vi "HEWH ANSI Get Rates.vi"(0 "ANSI Rate in":T3, 1 "Test Type - Rate":string(combo)="Rate", 5 "CO CO2 Data Array":string[][](array[string]), 7 "Gas Measurment Data":T2, 9 "Inficon Data - ALL":T1, 11 "error in (no error)":errorcluster, 12 "Software Elapsed Time":dbl format="%<%H:%M:%S>t") -> (3 "ANSI Display 1":string, 4 "ANSI Rate out":T3, 8 "Rate Outputs":string[][](array[string]), 14 "Test Complete":bool, 15 "error out":errorcluster)   [LabVIEW 2020]
uses:
  HEWH ANSI Rate.ctl
  Drivers/Alicat LabVIEW Drivers 2v1/Sub-VIs/Data Cluster.ctl
  Drivers/Inficon Transmitter/Type Definitions/Inficon Data.ctl
panel:
  out "Raw Timer Output":dbl format="%<%H:%M:%S>t"
  # "Natural Gas"
  # "Propane"
  # "Totalizer Timer"
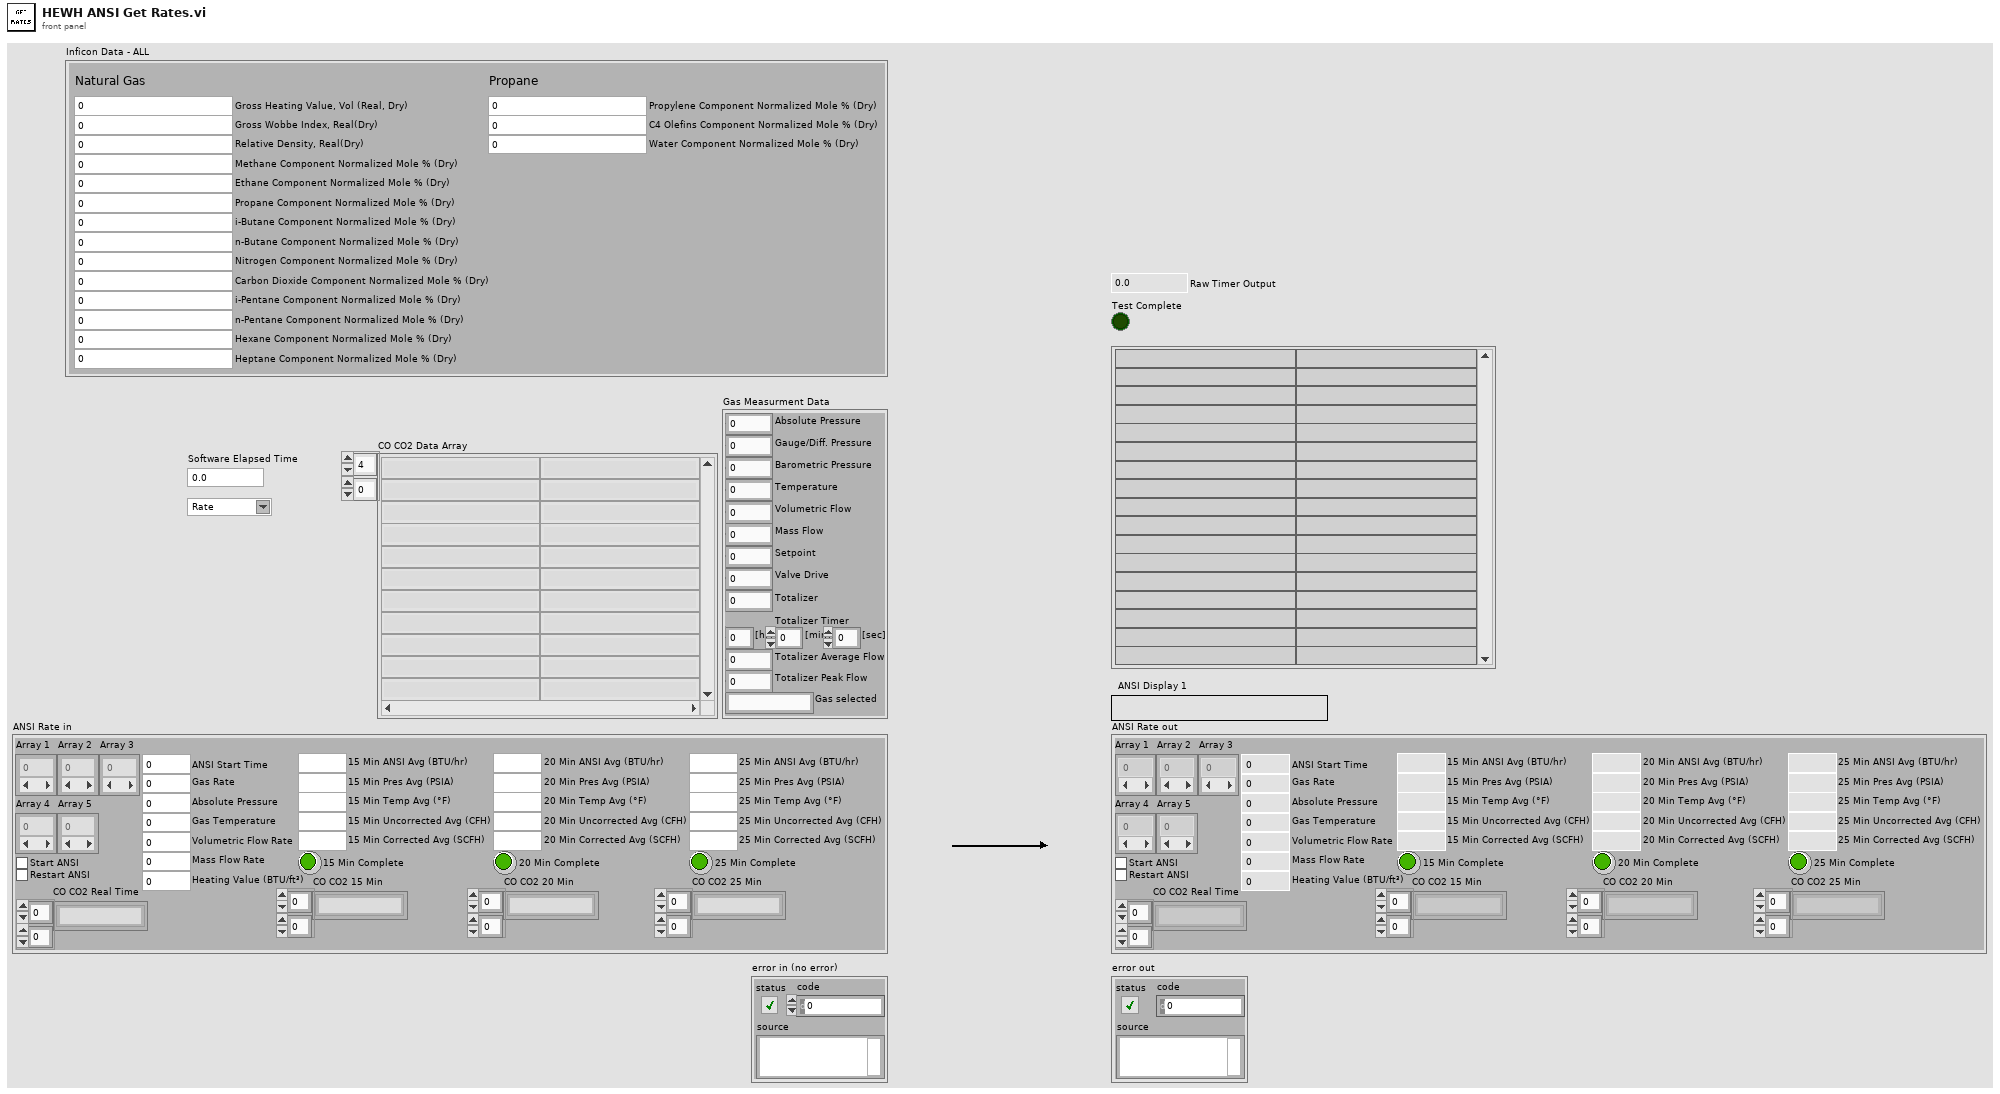
[diagram p1: front panel]
types:
  T1 = typedef "Inficon Data.ctl" = cluster{"Gross Heating Value, Vol (Real, Dry)":dbl, "Nitrogen Component Normalized Mole % (Dry)":dbl, "Methane Component Normalized Mole % (Dry)":dbl, "Carbon Dioxide Component Normalized Mole % (Dry)":dbl, "Ethane Component Normalized Mole % (Dry)":dbl, "Propane Component Normalized Mole % (Dry)":dbl, "i-Pentane Component Normalized Mole % (Dry)":dbl, "i-Butane Component Normalized Mole % (Dry)":dbl, "n-Butane Component Normalized Mole % (Dry)":dbl, "n-Pentane Component Normalized Mole % (Dry)":dbl, "Hexane Component Normalized Mole % (Dry)":dbl, "Heptane Component Normalized Mole % (Dry)":dbl, "Gross Wobbe Index, Real(Dry)":dbl, "Relative Density, Real(Dry)":dbl, "Propylene Component Normalized Mole % (Dry)":dbl, "C4 Olefins Component Normalized Mole % (Dry)":dbl, "Water Component Normalized Mole % (Dry)":dbl}
  T2 = typedef "Data Cluster.ctl" = cluster{"Absolute Pressure":dbl, "Gauge/Diff. Pressure":dbl, "Barometric Pressure":dbl, "Temperature":dbl, "Volumetric Flow":dbl, "Mass Flow":dbl, "Setpoint":dbl, "Valve Drive":dbl, "Totalizer":dbl, "[hr]":dbl, "[min]":dbl, "[sec]":dbl, "Totalizer Average Flow":dbl, "Totalizer Peak Flow":dbl, "Gas selected":string}
  T3 = typedef "HEWH ANSI Rate.ctl" = cluster{"Array 1":dbl[], "Array 3":dbl[], "Array 2":dbl[], "Start ANSI":bool, "ANSI Start Time":dbl, "Restart ANSI":bool, "15 Min ANSI Avg (BTU/hr)":dbl, "20 Min ANSI Avg (BTU/hr)":dbl, "25 Min ANSI Avg (BTU/hr)":dbl, "Absolute Pressure":dbl, "Gas Temperature":dbl, "Volumetric Flow Rate":dbl, "Mass Flow Rate":dbl, "Array 4":dbl[], "Array 5":dbl[], "Gas Rate":dbl, "15 Min Pres Avg (PSIA)":dbl, "20 Min Pres Avg (PSIA)":dbl, "25 Min Pres Avg (PSIA)":dbl, "15 Min Temp Avg (°F) ":dbl, "20 Min Temp Avg (°F)":dbl, "25 Min Temp Avg (°F)":dbl, "15 Min Uncorrected Avg (CFH)":dbl, "20 Min Uncorrected Avg (CFH)":dbl, "25 Min Uncorrected Avg (CFH)":dbl, "15 Min Corrected Avg (SCFH)":dbl, "20 Min Corrected Avg (SCFH)":dbl, "25 Min Corrected Avg (SCFH)":dbl, "15 Min Complete":bool, "20 Min Complete":bool, "25 Min Complete":bool, "Heating Value (BTU/ft³)":dbl, "CO CO2 15 Min":string[][], "CO CO2 20 Min":string[][], "CO CO2 25 Min":string[][], "CO CO2 Real Time":string[][]}
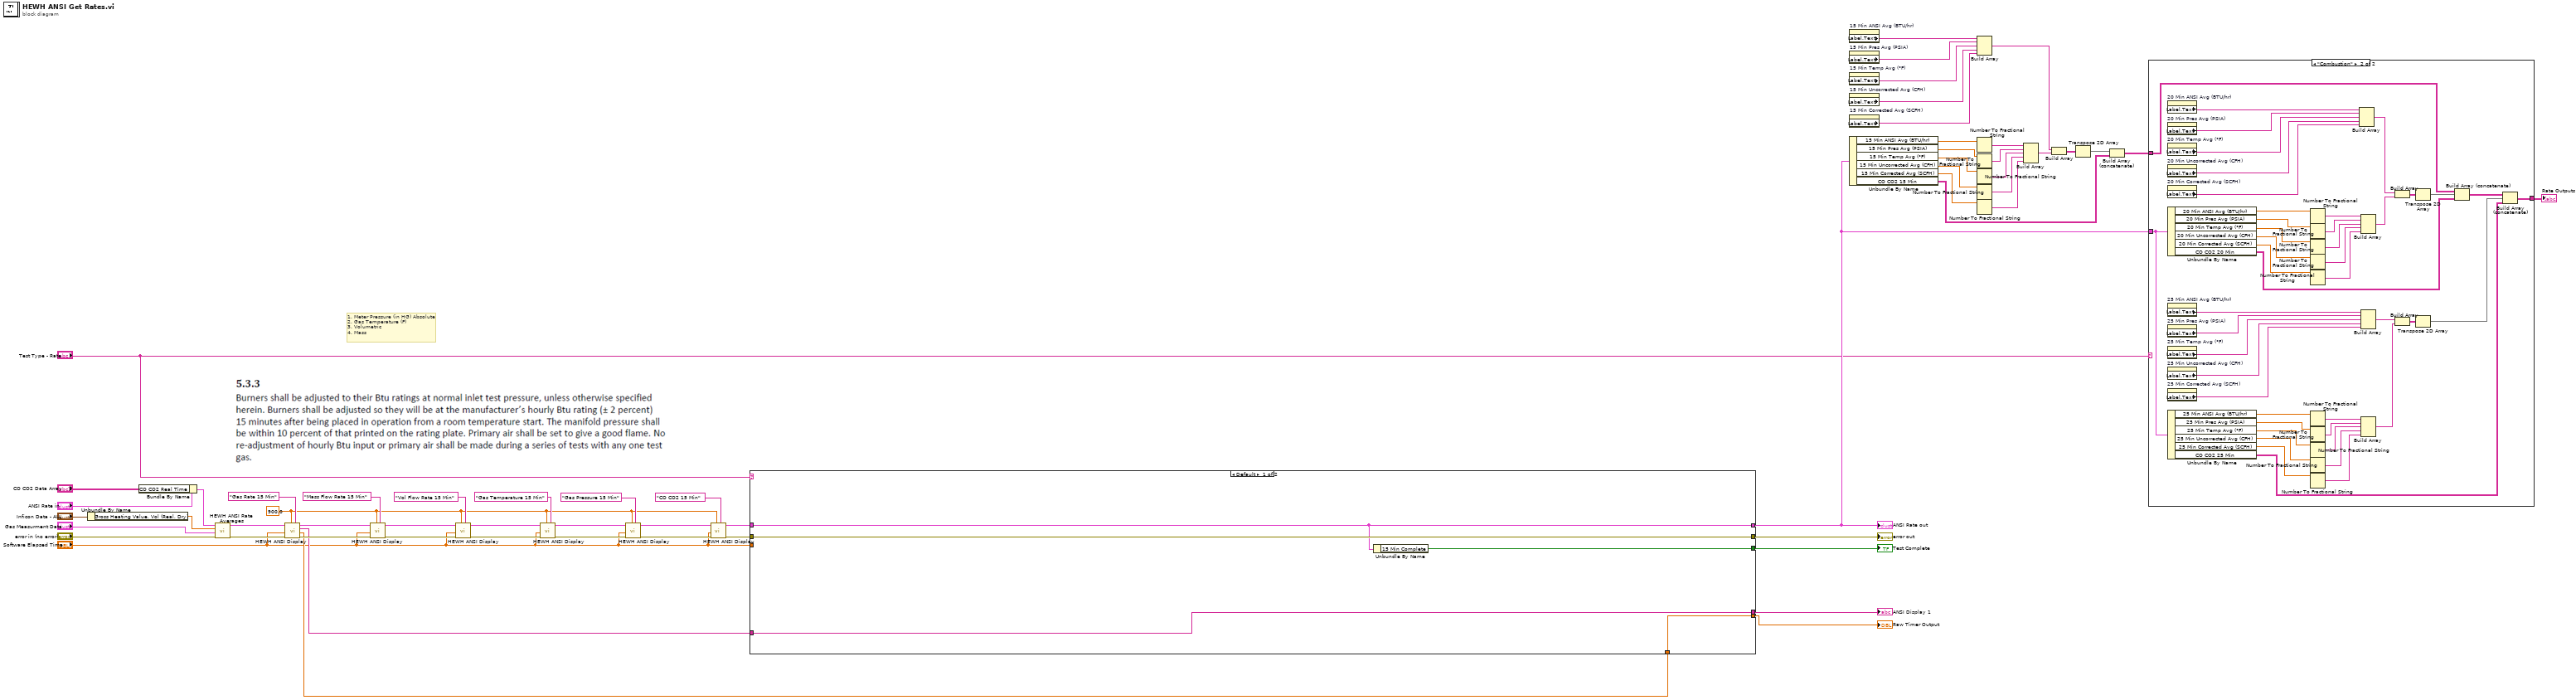
[diagram p0: block diagram]
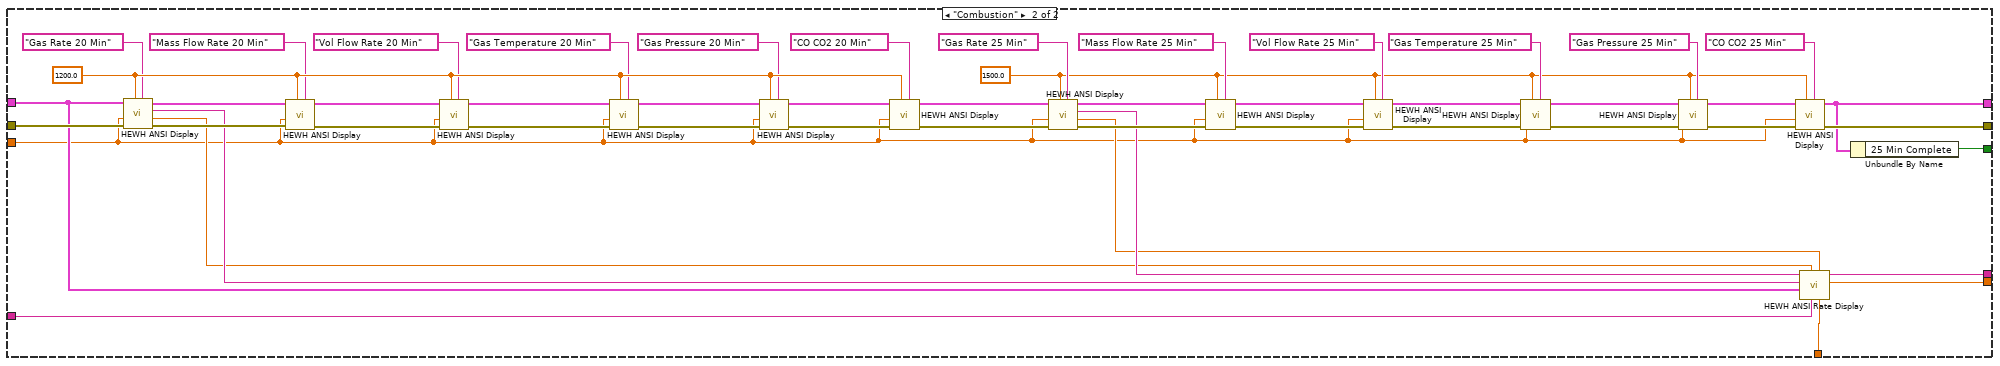
[diagram p3: hidden frame]
diagram:
  w11 = 900.0 ("Stop Timer")
  # "1. Meter Pressure (in HG) Absolute\n2. Gas Temperature (F)\n3. Volumetric\n4. Mass"
  n1 = Unbundle By Name("Inficon Data - ALL") -> ("Gross Heating Value, Vol (Real, Dry)"=w1:dbl)
  n2 = Bundle By Name(cluster="ANSI Rate in", "CO CO2 Real Time"="CO CO2 Data Array") -> (w9:T3)
  n3 = call "HEWH ANSI Rate Averages.vi"("error in (no error)"="error in (no error)", "Gas Measurment Data"="Gas Measurment Data", "Gross Heating Value, Vol (Real, Dry)"=w1, "ANSI Rate in"=w9) -> ("error out"=w57:errorcluster, "ANSI Rate out"=w56:T3)  [unwired: 6 in]
  n4 = call "HEWH ANSI Display.vi"("Calculation Type"="Gas Rate 15 Min", "Stop Timer"=w11, "Error In"=w57, "Software Elapsed Time"="Software Elapsed Time", "ANSI Rate In"=w56) -> ("Error Out"=w51:errorcluster, "Raw Timer"=w22:dbl, "ANSI Display"=w24:string, "ANSI Rate Out"=w55:T3)  [unwired: 3 in]
  n5 = call "HEWH ANSI Display.vi"("Calculation Type"="Mass Flow Rate 15 Min", "Stop Timer"=w11, "Error In"=w51, "Software Elapsed Time"="Software Elapsed Time", "ANSI Rate In"=w55) -> ("Error Out"=w50:errorcluster, "ANSI Rate Out"=w54:T3)  [unwired: 3 in, 2 out]
  n6 = call "HEWH ANSI Display.vi"("Calculation Type"="Vol Flow Rate 15 Min", "Stop Timer"=w11, "Error In"=w50, "Software Elapsed Time"="Software Elapsed Time", "ANSI Rate In"=w54) -> ("Error Out"=w49:errorcluster, "ANSI Rate Out"=w53:T3)  [unwired: 3 in, 2 out]
  n7 = call "HEWH ANSI Display.vi"("Calculation Type"="Gas Temperature 15 Min", "Stop Timer"=w11, "Error In"=w49, "Software Elapsed Time"="Software Elapsed Time", "ANSI Rate In"=w53) -> ("Error Out"=w48:errorcluster, "ANSI Rate Out"=w52:T3)  [unwired: 3 in, 2 out]
  n8 = call "HEWH ANSI Display.vi"("Calculation Type"="Gas Pressure 15 Min", "Stop Timer"=w11, "Error In"=w48, "Software Elapsed Time"="Software Elapsed Time", "ANSI Rate In"=w52) -> ("Error Out"=w13:errorcluster, "ANSI Rate Out"=w15:T3)  [unwired: 3 in, 2 out]
  n9 = call "HEWH ANSI Display.vi"("Calculation Type"="CO CO2 15 Min", "Stop Timer"=w11, "Error In"=w13, "Software Elapsed Time"="Software Elapsed Time", "ANSI Rate In"=w15) -> ("Error Out"=w12:errorcluster, "ANSI Rate Out"=w14:T3)  [unwired: 3 in, 2 out]
  n10 = case shown="Default" "Test Type - Rate" {
    tunnel: w12 -> [w64 w114]
    tunnel: w14 -> [w63 w96]
    tunnel: [w64 w70] -> w47
    tunnel: [w63 w68] -> w46
    tunnel: "Software Elapsed Time" -> [_ w66]
    tunnel: [w62 w97] -> w25
    tunnel: w24 -> [w61 w95]
    tunnel: [w61 w94] -> w23
    tunnel: w22 -> [w60 w91]
    tunnel: [w60 w88] -> w3
    frame Default {
      n11 = Unbundle By Name(w63) -> ("15 Min Complete"=w62:bool)
    }
    frame "Combustion" {
      w67 = 1500.0 ("Stop Timer")
      w82 = 1200.0 ("Stop Timer")
      n12 = call "HEWH ANSI Display.vi"("Calculation Type"="Gas Rate 20 Min", "Stop Timer"=w82, "Error In"=w114, "Software Elapsed Time"=w66, "ANSI Rate In"=w96) -> ("Error Out"=w113:errorcluster, "Raw Timer"=w90:dbl, "ANSI Display"=w93:string, "ANSI Rate Out"=w106:T3)  [unwired: 3 in]
      n13 = call "HEWH ANSI Display.vi"("Calculation Type"="Mass Flow Rate 20 Min", "Stop Timer"=w82, "Error In"=w113, "Software Elapsed Time"=w66, "ANSI Rate In"=w106) -> ("Error Out"=w112:errorcluster, "ANSI Rate Out"=w107:T3)  [unwired: 3 in, 2 out]
      n14 = call "HEWH ANSI Display.vi"("Calculation Type"="Vol Flow Rate 20 Min", "Stop Timer"=w82, "Error In"=w112, "Software Elapsed Time"=w66, "ANSI Rate In"=w107) -> ("Error Out"=w111:errorcluster, "ANSI Rate Out"=w108:T3)  [unwired: 3 in, 2 out]
      n15 = call "HEWH ANSI Display.vi"("Calculation Type"="Gas Temperature 20 Min", "Stop Timer"=w82, "Error In"=w111, "Software Elapsed Time"=w66, "ANSI Rate In"=w108) -> ("Error Out"=w110:errorcluster, "ANSI Rate Out"=w109:T3)  [unwired: 3 in, 2 out]
      n16 = call "HEWH ANSI Display.vi"("Calculation Type"="Gas Pressure 20 Min", "Stop Timer"=w82, "Error In"=w110, "Software Elapsed Time"=w66, "ANSI Rate In"=w109) -> ("Error Out"=w84:errorcluster, "ANSI Rate Out"=w87:T3)  [unwired: 3 in, 2 out]
      n17 = call "HEWH ANSI Display.vi"("Calculation Type"="CO CO2 20 Min", "Stop Timer"=w82, "Error In"=w84, "Software Elapsed Time"=w66, "ANSI Rate In"=w87) -> ("Error Out"=w83:errorcluster, "ANSI Rate Out"=w86:T3)  [unwired: 3 in, 2 out]
      n18 = call "HEWH ANSI Display.vi"("Calculation Type"="Gas Rate 25 Min", "Stop Timer"=w67, "Error In"=w83, "Software Elapsed Time"=w66, "ANSI Rate In"=w86) -> ("Error Out"=w105:errorcluster, "Raw Timer"=w89:dbl, "ANSI Display"=w92:string, "ANSI Rate Out"=w101:T3)  [unwired: 3 in]
      n19 = call "HEWH ANSI Display.vi"("Calculation Type"="Mass Flow Rate 25 Min", "Stop Timer"=w67, "Error In"=w105, "Software Elapsed Time"=w66, "ANSI Rate In"=w101) -> ("Error Out"=w104:errorcluster, "ANSI Rate Out"=w100:T3)  [unwired: 3 in, 2 out]
      n20 = call "HEWH ANSI Display.vi"("Calculation Type"="Vol Flow Rate 25 Min", "Stop Timer"=w67, "Error In"=w104, "Software Elapsed Time"=w66, "ANSI Rate In"=w100) -> ("Error Out"=w103:errorcluster, "ANSI Rate Out"=w99:T3)  [unwired: 3 in, 2 out]
      n21 = call "HEWH ANSI Display.vi"("Calculation Type"="Gas Temperature 25 Min", "Stop Timer"=w67, "Error In"=w103, "Software Elapsed Time"=w66, "ANSI Rate In"=w99) -> ("Error Out"=w102:errorcluster, "ANSI Rate Out"=w98:T3)  [unwired: 3 in, 2 out]
      n22 = call "HEWH ANSI Display.vi"("Calculation Type"="Gas Pressure 25 Min", "Stop Timer"=w67, "Error In"=w102, "Software Elapsed Time"=w66, "ANSI Rate In"=w98) -> ("Error Out"=w71:errorcluster, "ANSI Rate Out"=w69:T3)  [unwired: 3 in, 2 out]
      n23 = call "HEWH ANSI Display.vi"("Calculation Type"="CO CO2 25 Min", "Stop Timer"=w67, "Error In"=w71, "Software Elapsed Time"=w66, "ANSI Rate In"=w69) -> ("Error Out"=w70:errorcluster, "ANSI Rate Out"=w68:T3)  [unwired: 3 in, 2 out]
      n24 = call "HEWH ANSI Rate Display.vi"("Raw Timer 15"=w91, "Raw Timer 25"=w89, "15 Min Display"=w95, "Raw Timer 20"=w90, "ANSI Rate Out"=w96, "20 Min Display"=w93, "25 Min Display"=w92) -> ("Raw Timer Output"=w88:dbl, "Output Display"=w94:string)  [unwired: 2 in, 1 out]
      n25 = Unbundle By Name(w68) -> ("25 Min Complete"=w97:bool)
    }
  }
  "ANSI Display 1" <- w23
  "ANSI Rate out" <- w46
  "error out" <- w47
  "Test Complete" <- w25
  "Raw Timer Output" <- w3
  n26 = property on="15 Min ANSI Avg (BTU/hr)" class="DigNum (strict)"() -> ("Label.Text"=w33:string)  [unwired: 2 in, 2 out]
  n27 = property on="15 Min Pres Avg (PSIA)" class="DigNum (strict)"() -> ("Label.Text"=w32:string)  [unwired: 2 in, 2 out]
  n28 = property on="15 Min Temp Avg (°F)" class="DigNum (strict)"() -> ("Label.Text"=w31:string)  [unwired: 2 in, 2 out]
  n29 = property on="15 Min Uncorrected Avg (CFH)" class="DigNum (strict)"() -> ("Label.Text"=w30:string)  [unwired: 2 in, 2 out]
  n30 = property on="15 Min Corrected Avg (SCFH)" class="DigNum (strict)"() -> ("Label.Text"=w29:string)  [unwired: 2 in, 2 out]
  n31 = Unbundle By Name(w46) -> ("15 Min ANSI Avg (BTU/hr)"=w45:dbl, "15 Min Pres Avg (PSIA)"=w43:dbl, "15 Min Temp Avg (°F)"=w41:dbl, "15 Min Uncorrected Avg (CFH)"=w39:dbl, "15 Min Corrected Avg (SCFH)"=w37:dbl, "CO CO2 15 Min"=w5:string[][])
  n32 = Build Array(w33, w32, w31, w30, w29) -> (w28:string[])
  n33 = Number To Fractional String(number=w45) -> (F-format string=w44:string)  [unwired: 3 in]
  n34 = Number To Fractional String(number=w43) -> (F-format string=w42:string)  [unwired: 3 in]
  n35 = Number To Fractional String(number=w41) -> (F-format string=w40:string)  [unwired: 3 in]
  n36 = Number To Fractional String(number=w39) -> (F-format string=w38:string)  [unwired: 3 in]
  n37 = Number To Fractional String(number=w37) -> (F-format string=w36:string)  [unwired: 3 in]
  n38 = Build Array(w44, w42, w40, w38, w36) -> (w35:string[])
  n39 = Build Array(w28, w35) -> (w34:string[][])
  n40 = Transpose 2D Array(2D array=w34) -> (transposed array=w7:string[][])
  n41 = Build Array (concatenate)(w7, w5) -> (w6:string[][])
  n42 = case shown="\"Combustion\"" "Test Type - Rate" {
    tunnel: w46 -> [_ w159]
    tunnel: [w115 w118] -> w26
    tunnel: w6 -> [w115 w134]
    frame Default {
    }
    frame "Combustion" {
      n43 = property on="20 Min ANSI Avg (BTU/hr)" class="DigNum (strict)"() -> ("Label.Text"=w148:string)  [unwired: 2 in, 2 out]
      n44 = property on="20 Min Pres Avg (PSIA)" class="DigNum (strict)"() -> ("Label.Text"=w147:string)  [unwired: 2 in, 2 out]
      n45 = property on="20 Min Temp Avg (°F)" class="DigNum (strict)"() -> ("Label.Text"=w146:string)  [unwired: 2 in, 2 out]
      n46 = property on="20 Min Uncorrected Avg (CFH)" class="DigNum (strict)"() -> ("Label.Text"=w145:string)  [unwired: 2 in, 2 out]
      n47 = property on="20 Min Corrected Avg (SCFH)" class="DigNum (strict)"() -> ("Label.Text"=w144:string)  [unwired: 2 in, 2 out]
      n48 = Unbundle By Name(w159) -> ("20 Min ANSI Avg (BTU/hr)"=w158:dbl, "20 Min Pres Avg (PSIA)"=w157:dbl, "20 Min Temp Avg (°F)"=w156:dbl, "20 Min Uncorrected Avg (CFH)"=w155:dbl, "20 Min Corrected Avg (SCFH)"=w154:dbl, "CO CO2 20 Min"=w128:string[][])
      n49 = property on="25 Min ANSI Avg (BTU/hr)" class="DigNum (strict)"() -> ("Label.Text"=w127:string)  [unwired: 2 in, 2 out]
      n50 = property on="25 Min Pres Avg (PSIA)" class="DigNum (strict)"() -> ("Label.Text"=w126:string)  [unwired: 2 in, 2 out]
      n51 = property on="25 Min Temp Avg (°F)" class="DigNum (strict)"() -> ("Label.Text"=w125:string)  [unwired: 2 in, 2 out]
      n52 = property on="25 Min Uncorrected Avg (CFH)" class="DigNum (strict)"() -> ("Label.Text"=w124:string)  [unwired: 2 in, 2 out]
      n53 = property on="25 Min Corrected Avg (SCFH)" class="DigNum (strict)"() -> ("Label.Text"=w123:string)  [unwired: 2 in, 2 out]
      n54 = Unbundle By Name(w159) -> ("25 Min ANSI Avg (BTU/hr)"=w153:dbl, "25 Min Pres Avg (PSIA)"=w152:dbl, "25 Min Temp Avg (°F)"=w151:dbl, "25 Min Uncorrected Avg (CFH)"=w150:dbl, "25 Min Corrected Avg (SCFH)"=w149:dbl, "CO CO2 25 Min"=w116:string[][])
      n55 = Number To Fractional String(number=w158) -> (F-format string=w143:string)  [unwired: 3 in]
      n56 = Number To Fractional String(number=w157) -> (F-format string=w142:string)  [unwired: 3 in]
      n57 = Number To Fractional String(number=w156) -> (F-format string=w141:string)  [unwired: 3 in]
      n58 = Number To Fractional String(number=w155) -> (F-format string=w140:string)  [unwired: 3 in]
      n59 = Number To Fractional String(number=w154) -> (F-format string=w139:string)  [unwired: 3 in]
      n60 = Number To Fractional String(number=w153) -> (F-format string=w133:string)  [unwired: 3 in]
      n61 = Number To Fractional String(number=w152) -> (F-format string=w132:string)  [unwired: 3 in]
      n62 = Number To Fractional String(number=w151) -> (F-format string=w131:string)  [unwired: 3 in]
      n63 = Number To Fractional String(number=w150) -> (F-format string=w130:string)  [unwired: 3 in]
      n64 = Number To Fractional String(number=w149) -> (F-format string=w129:string)  [unwired: 3 in]
      n65 = Build Array(w148, w147, w146, w145, w144) -> (w137:string[])
      n66 = Build Array(w143, w142, w141, w140, w139) -> (w136:string[])
      n67 = Build Array(w127, w126, w125, w124, w123) -> (w121:string[])
      n68 = Build Array(w133, w132, w131, w130, w129) -> (w120:string[])
      n69 = Build Array(w137, w136) -> (w138:string[][])
      n70 = Build Array(w121, w120) -> (w122:string[][])
      n71 = Transpose 2D Array(2D array=w138) -> (transposed array=w135:string[][])
      n72 = Transpose 2D Array(2D array=w122) -> (transposed array=w117:string[][])
      n73 = Build Array (concatenate)(w134, w135, w128) -> (w119:string[][])
      n74 = Build Array (concatenate)(w119, w117, w116) -> (w118:string[][])
    }
  }
  "Rate Outputs" <- w26
